vi "Main.vi"() -> ()   [LabVIEW 2019]
doc: "Use this template to build a simple state machine design pattern. Each state executes code and determines which state to transition to."
uses:
  controls/State.ctl
  controls/Data.ctl
  19129ee7-2167-46f5-94c7-6c94359de5af.vi
  97020e74-c88b-4e28-9d88-861c136ab0ec.vi
  3c8d42af-6aab-4c71-abb2-08a78789fadc.vi
  e1166f26-e34e-4867-bf64-0f2b722d0543.vi
  bf01d7cc-2561-4f26-92a1-0952a6f05fec.vi
  86db6c87-178c-447d-b6dd-f69cb95457e9.vi
  da4ff3ae-118d-429f-89dd-6d204435764b.vi
  6bd7f036-247f-456b-9d75-44be66b4905f.vi
  945257d8-b946-4064-894d-b06f0ac42300.vi
  0b4e00a9-1667-44d7-8672-90e7e78b343c.vi
  5caef232-9b1d-433d-a0d0-0ef1dc360dc2.vi
  663dc032-b822-4887-a4ac-48573fd9169f.vi
  31c5358b-7e5d-432a-9607-e566ad1521c2.vi
  71a76362-c902-4af5-9e49-a2a977d014ca.vi
  ba676aeb-3a27-434e-9a7e-9afe782587b5.vi
  86c68439-f49f-4d4b-9d68-38f5b6fe5469.vi
  25f27556-7067-46a7-b570-d4658504531b.vi
  eab5cf03-8b77-4dda-81a4-4f254e97d93e.vi
  fdccc99e-0b2a-4617-a728-f0ef31699cf6.vi
  a5814f98-bddc-4bba-a6ba-c09daa687ff9.vi
panel:
  out "Cycle":u64
  out "Result":bool
  out "LED_OFF":bool
  out "LED_ON":bool
  out "Fan_On (rpm)":dbl
  out "FAN_OFF":bool
  out "FAN_ON":bool
  out "Time_Out":i8
  out "Status":string
  out "Motor_Lock":bool
  out "CAN_ID":u32 format="%.0x"
  out "Motor_Unlock":bool
  out "Rx_DATA":u8[](array[numeric]) format="%x"
  in  "Rx_ID":u32=1968
  out "Tx_DATA":u8[](array[numeric])
  out "Tx_ID":u32=1952
  out "CAN_Tx":bool
  in  "Stop":bool
  in  "TPCANMsg To Write":T1 {"ID" format="%x"; "MSGTYPE" items=["STATUS"=128, "EXTENDED"=2, "RTR"=1, "DATA MSG"=0]; "aDATA" format="%x"}
  out "Last Error":string
  in  "Start":bool
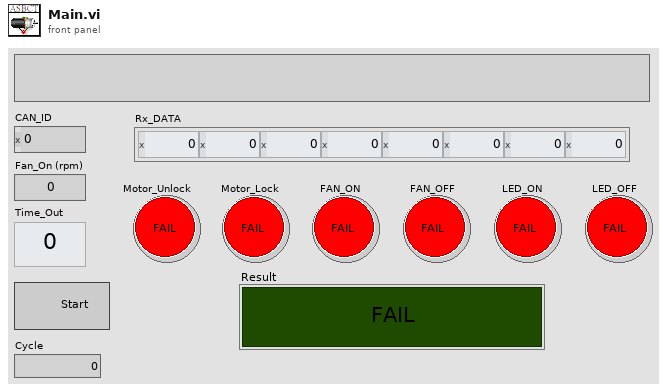
[diagram p1: front panel]
types:
  T1 = cluster{"ID":u32, "MSGTYPE":u8, "LEN":u8, "aDATA":u8[]}
  T2 = typedef "Data.ctl" = cluster{"Status":string, "Cycle":u64, "Result":bool[]}
  T3 = typedef "State.ctl" = enum16{"Initialize", "Wait for Event", "Motor_Remove", "Motor_Insert", "Fan_On", "Fan_Off", "Led_On", "Led_Off"}
  T4 = typedef "PCAN_ERROR.ctl" = i32
  T5 = cluster{"Is Warning":bool, "Is Error":bool, "Message":string}
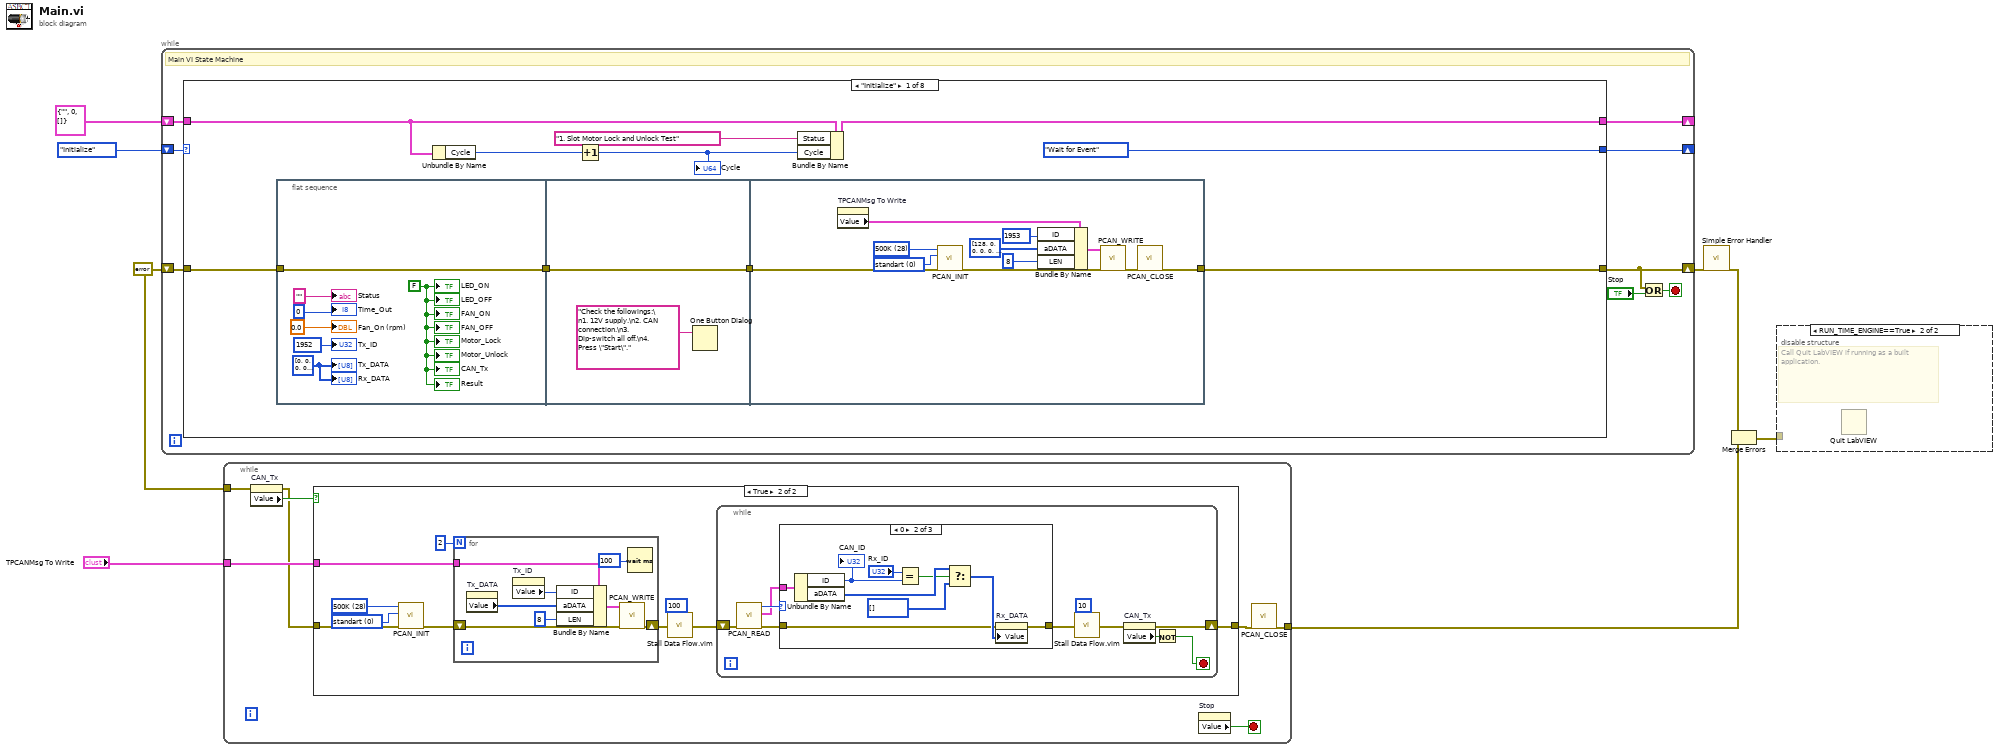
[diagram p0: block diagram]
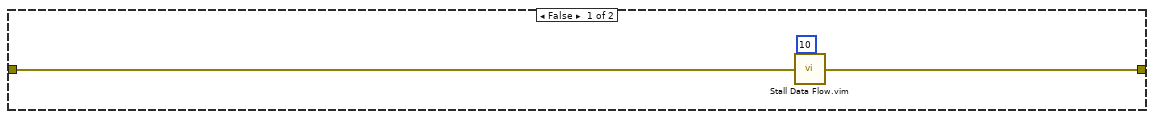
[diagram p2: hidden frame]
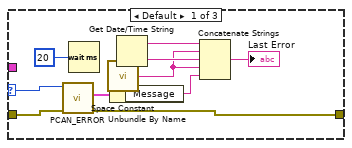
[diagram p3: hidden frame]
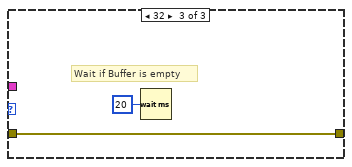
[diagram p4: hidden frame]
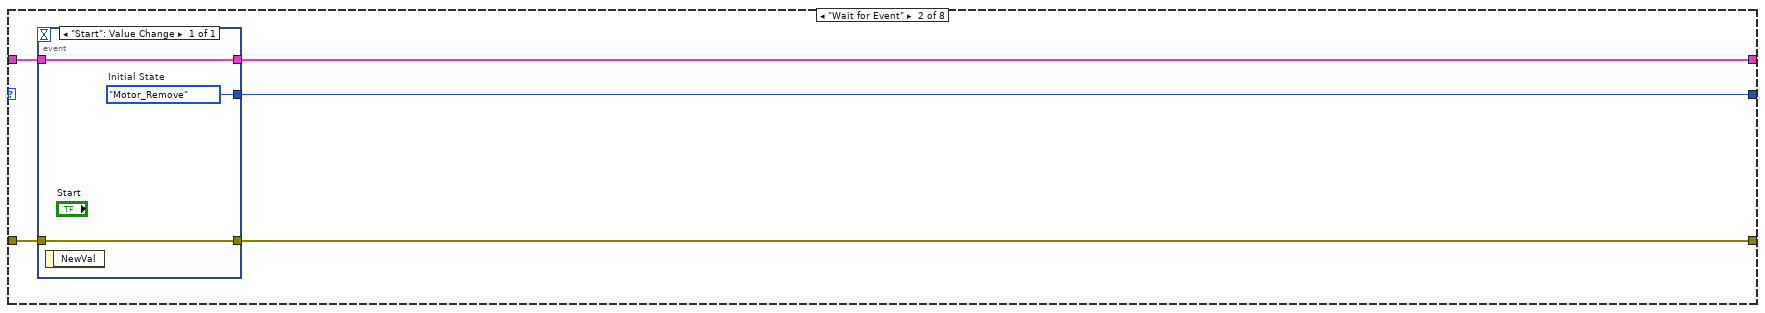
[diagram p6: hidden frame]
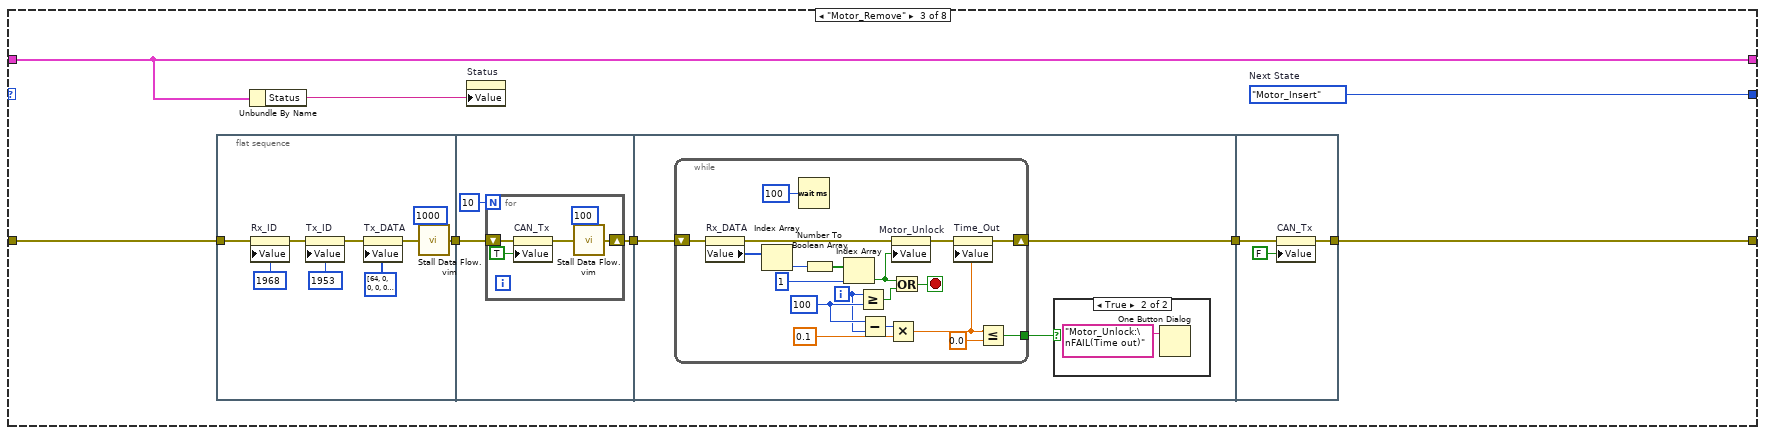
[diagram p7: hidden frame]
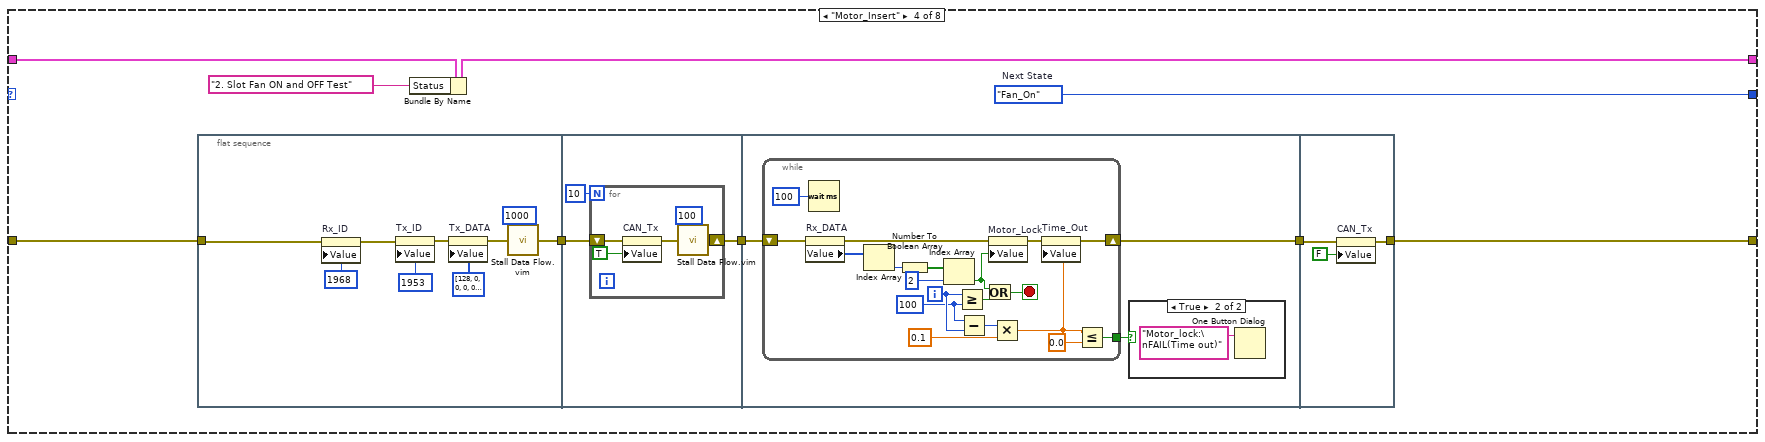
[diagram p9: hidden frame]
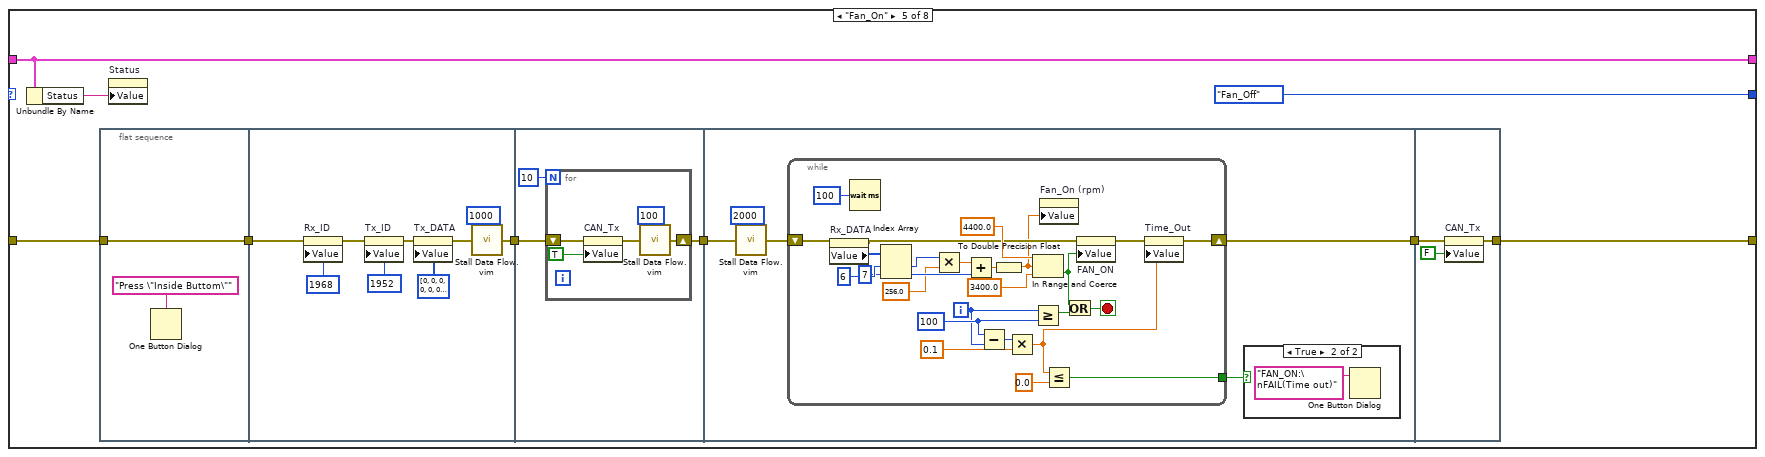
[diagram p11: hidden frame]
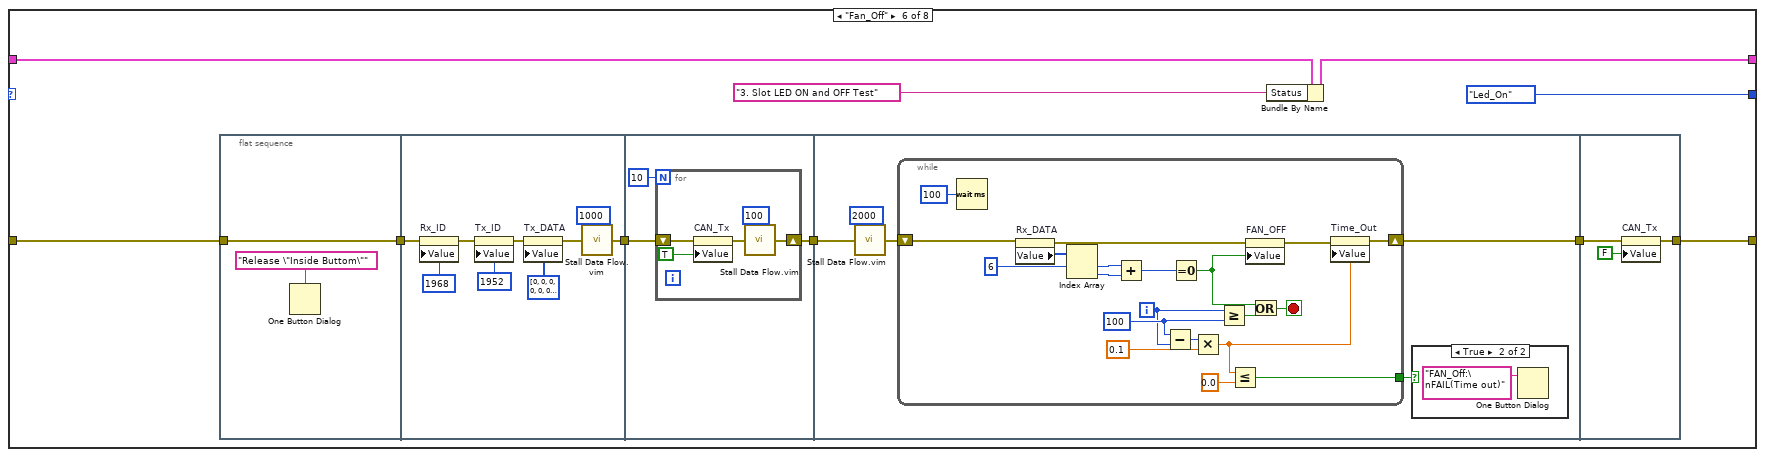
[diagram p13: hidden frame]
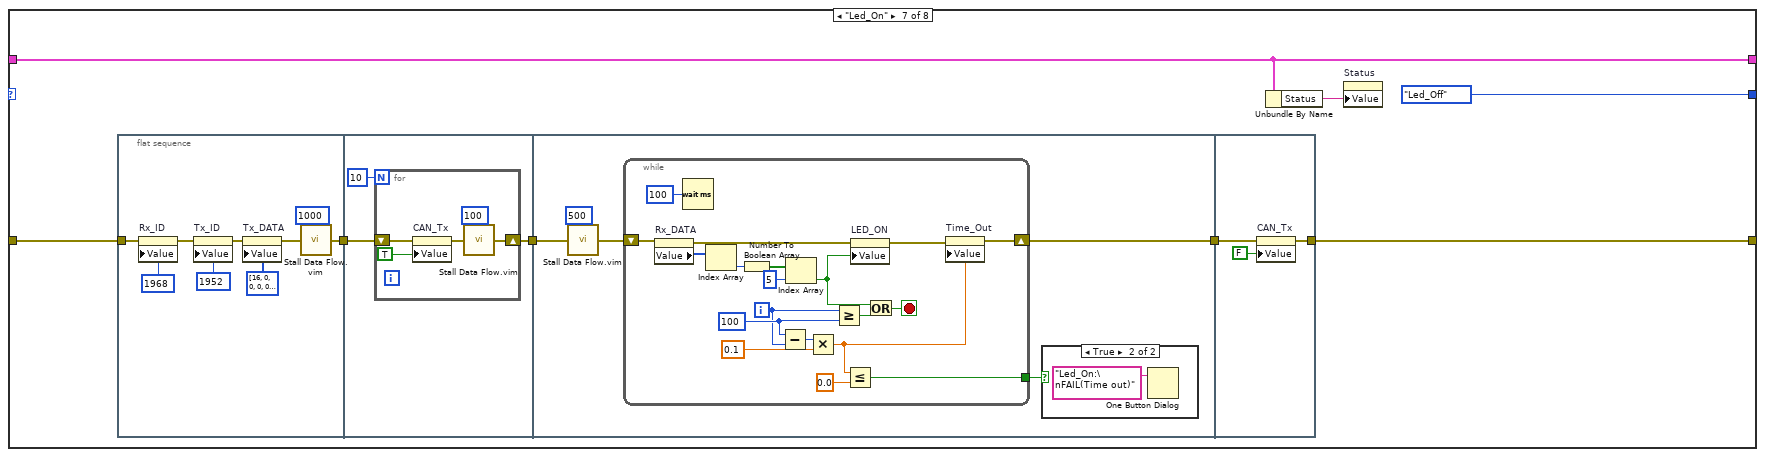
[diagram p15: hidden frame]
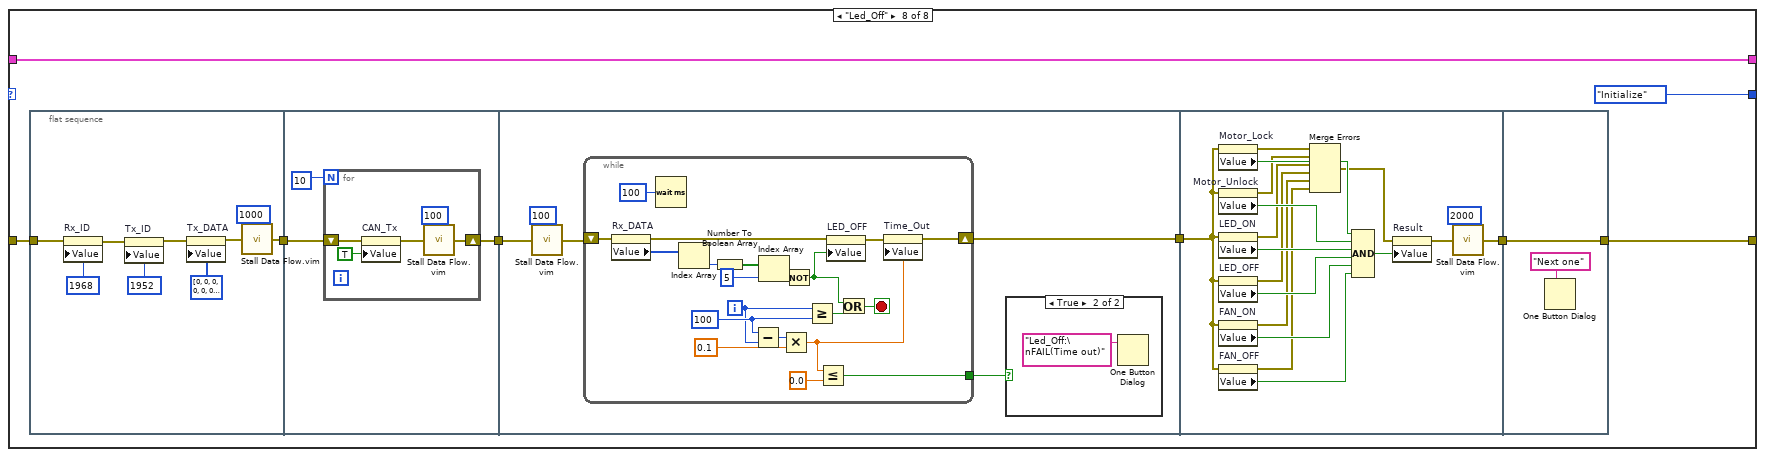
[diagram p17: hidden frame]
diagram:
  w1 = errorcluster {"status"=FALSE, "code"=0, "source"=""} ("error constant")
  n1 = while {
    shift-right: [w10] -> _
    shift-left: State."Initialize" ("Initial State") -> [w11]
    shift-right: [w15] -> _
    shift-left: T2 {"Status"="", "Cycle"=0, "Result"=[]} ("Data") -> [w16]
    shift-right: [w12] -> w7
    shift-left: w1 -> [w14]
    stop <- w13 stop-if-true
    # "Main VI State Machine"
    n2 = case shown="\"Initialize\"" w11 {
      tunnel: [State."Wait for Event" ("Next") w47 w62 w114 State."Fan_Off" ("(Value Not Used)") State."Led_On" ("(Value Not Used)") State."Led_Off" ("(Value Not Used)") State."Initialize" ("(Value Not Used)")] -> w10
      tunnel: w16 -> [w19 w51 w60 w111 w162 w225 w280 w332]
      tunnel: [w26 w50 w60 w110 w162 w224 w280 w332] -> w15
      tunnel: w14 -> [w23 w49 w61 w112 w164 w228 w284 w337]
      tunnel: [w24 w48 w55 w106 w158 w222 w281 w338] -> w12
      frame "Initialize" {
        # "Initialize - Initialize the application."
        n3 = flat-sequence {
          tunnel: w23 -> [w33]
          tunnel: [w33] -> w21
          tunnel: w21 -> [w35]
          tunnel: [w35] -> w20
          tunnel: [w36] -> w24
          tunnel: w20 -> [w44]
          frame #0 {
            w28 = u8[] [0, 0, 0, 0, 0, 0, 0, 0] ("aDATA")
            w27 = FALSE ("Replace_Me_Boolean")
            "Time_Out" <- i8 0 ("Time_Out")
            "Status" <- "" ("Status")
            "Fan_On (rpm)" <- 0.0 ("FAN(rpm)")
            "CAN_Tx" <- w27
            "Motor_Unlock" <- w27
            "Motor_Lock" <- w27
            "FAN_ON" <- w27
            "FAN_OFF" <- w27
            "LED_ON" <- w27
            "LED_OFF" <- w27
            "Tx_ID" <- u32 1952 ("ID")
            "Tx_DATA" <- w28
            "Rx_DATA" <- w28
            "Result" <- w27
          }
          frame #1 {
            n4 = One Button Dialog(message="Check the followings:\n1. 12V supply.\n2. CAN connection.\n3. Dip-switch all off.\n4. Press \"Start\".") -> ()  [unwired: 1 in, 1 out]
          }
          frame #2 {
            w46 = 0 items=["standart", "extended"] ("type")
            w45 = u16 28 items=["1M"=20, "500K"=28, "250K"=284, "125K"=796, "100K"=17199, "50K"=18223, "20K"=21295, "10K"=26415, "5K"=32639] ("baud")
            n5 = property on="TPCANMsg To Write" class="Clust (strict)"() -> ("Value"=w42:T1)  [unwired: 2 in, 2 out]
            n6 = call "PCAN_INIT.vi"("error in (no error)"=w44, "Msg Type"=w46, "BTR0BTR1"=w45) -> ("error out"=w40:errorcluster)  [unwired: 1 in, 7 out]
            n7 = Bundle By Name(cluster=w42, "ID"=u32 1953, "aDATA"=u8[] [128, 0, 0, 0, 0, 0, 0, 0], "LEN"=u8 8) -> (w41:T1)
            n8 = call "PCAN_WRITE.vi"("error in (no error)"=w40, "TPCANMsg"=w41) -> ("error out"=w37:errorcluster)  [unwired: 1 in, 8 out]
            n9 = call "PCAN_CLOSE.vi"("error in (no error)"=w37) -> ("error out"=w36:errorcluster)  [unwired: 10 out]
          }
        }
        n10 = Unbundle By Name(w19) -> ("Cycle"=w18:u64)
        n11 = Increment(x=w18) -> (x+1=w17:u64)
        "Cycle" <- w17
        n12 = Bundle By Name(cluster=w19, "Status"="1. Slot Motor Lock and Unlock Test" ("Running User State 1"), "Cycle"=w17) -> (w26:T2)
      }
      frame "Wait for Event" {
        # "Wait for Event - Use an Event Structure to monitor the user interface for events that run different states of the state machine."
        n13 = event shown="[0] \"Start\": Value Change" {
          selector: _ -> [_]
          dyn-events: _ -> [_]
          timeout: _ -> [_]
          tunnel: [w53] -> w47
          tunnel: w51 -> [w52]
          tunnel: [w52] -> w50
          tunnel: w49 -> [w54]
          tunnel: [w54] -> w48
          event "Start": Value Change {
            w53 = State."Motor_Remove"  # Initial State
            n14 = event-data() -> ()  [unwired: 1 in, 1 out]
          }
        }
      }
      frame "Motor_Remove" {
        w62 = State."Motor_Insert"  # Next State
        # "User State 1 - Replace this state with functionality for your own application."
        n15 = flat-sequence {
          tunnel: w61 -> [w63]
          tunnel: [w66] -> w57
          tunnel: w57 -> [w74]
          tunnel: [w72] -> w56
          tunnel: [w82] -> w58
          tunnel: w56 -> [w80]
          tunnel: [w104] -> w55
          tunnel: w58 -> [w105]
          frame #0 {
            n16 = property on="Rx_ID" class="DigNum (strict)"(error in=w63, "Value"=u32 1968 ("Rx_ID")) -> (error out=w64:errorcluster)  [unwired: 1 in, 1 out]
            n17 = property on="Tx_ID" class="DigNum (strict)"(error in=w64, "Value"=u32 1953 ("ID")) -> (error out=w69:errorcluster)  [unwired: 1 in, 1 out]
            n18 = property on="Tx_DATA" class="Arr (strict)"(error in=w69, "Value"=u8[] [64, 0, 0, 0, 0, 0, 0, 0] ("aDATA")) -> (error out=w67:errorcluster)  [unwired: 1 in, 1 out]
            n19 = call "Stall Data Flow.vim"("value in"=w67, "milliseconds to wait"=u32 1000) -> ("value out"=w66:errorcluster)  [unwired: 1 out]
          }
          frame #1 {
            n20 = for {
              N: 10 -> [_]
              shift-right: [w76] -> w72
              shift-left: w74 -> [w79]
              n21 = property on="CAN_Tx" class="Bool (strict)"(error in=w79, "Value"=TRUE ("CAN_Tx")) -> (error out=w75:errorcluster)  [unwired: 1 in, 1 out]
              n22 = call "Stall Data Flow.vim"("value in"=w75, "milliseconds to wait"=u32 100) -> ("value out"=w76:errorcluster)  [unwired: 1 out]
            }
          }
          frame #2 {
            n23 = while {
              shift-right: [w92] -> w82
              shift-left: w80 -> [w88]
              tunnel: [w89] -> w81
              i -> [w96]
              stop <- w98 stop-if-true
              w97 = 100
              n24 = property on="Rx_DATA" class="Arr (strict)"(error in=w88) -> (error out=w100:errorcluster, "Value"=w102:u8[])  [unwired: 1 in, 1 out]
              n25 = Index Array(array=w102) -> (element=w85:u8)  [unwired: 1 in]
              n26 = Wait (ms)(milliseconds to wait=u32 100) -> ()  [unwired: 1 out]
              n27 = Number To Boolean Array(number=w85) -> (Boolean array=w86:bool[])
              n28 = Index Array(array=w86, index=1) -> (element=w84:bool)
              n29 = Greater Or Equal?(x=w96, y=w97) -> (x >= y?=w99:bool)
              n30 = Subtract(x=w97, y=w96) -> (x-y=w95:i32)
              n31 = Multiply(x=w95, y=0.1) -> (x*y=w91:dbl)
              n32 = property on="Motor_Unlock" class="Bool (strict)"(error in=w100, "Value"=w84) -> (error out=w93:errorcluster)  [unwired: 1 in, 1 out]
              n33 = Or(x=w84, y=w99) -> (x .or. y?=w98:bool)
              n34 = property on="Time_Out" class="DigNum (strict)"(error in=w93, "Value"=w91) -> (error out=w92:errorcluster)  [unwired: 1 in, 1 out]
              n35 = Less Or Equal?(x=w91, y=0.0) -> (x <= y?=w89:bool)
            }
            n36 = case shown="True" w81 {
              frame False {
              }
              frame True {
                n37 = One Button Dialog(message="Motor_Unlock:\nFAIL(Time out)") -> ()  [unwired: 1 in, 1 out]
              }
            }
          }
          frame #3 {
            n38 = property on="CAN_Tx" class="Bool (strict)"(error in=w105, "Value"=FALSE ("CAN_Tx")) -> (error out=w104:errorcluster)  [unwired: 1 in, 1 out]
          }
        }
        n39 = Unbundle By Name(w60) -> ("Status"=w59:string)
        n40 = property on="Status" class="Str"("Value"=w59) -> ()  [unwired: 2 in, 2 out]
      }
      frame "Motor_Insert" {
        w114 = State."Fan_On"  # Next State
        # "User State 2 - Replace this state with functionality for your own application."
        n41 = flat-sequence {
          tunnel: w112 -> [w115]
          tunnel: [w118] -> w113
          tunnel: w113 -> [w126]
          tunnel: [w124] -> w107
          tunnel: [w134] -> w108
          tunnel: w107 -> [w132]
          tunnel: [w156] -> w106
          tunnel: w108 -> [w157]
          frame #0 {
            n42 = property on="Rx_ID" class="DigNum (strict)"(error in=w115, "Value"=u32 1968 ("Rx_ID")) -> (error out=w116:errorcluster)  [unwired: 1 in, 1 out]
            n43 = property on="Tx_ID" class="DigNum (strict)"(error in=w116, "Value"=u32 1953 ("ID")) -> (error out=w121:errorcluster)  [unwired: 1 in, 1 out]
            n44 = property on="Tx_DATA" class="Arr (strict)"(error in=w121, "Value"=u8[] [128, 0, 0, 0, 0, 0, 0, 0] ("aDATA")) -> (error out=w119:errorcluster)  [unwired: 1 in, 1 out]
            n45 = call "Stall Data Flow.vim"("value in"=w119, "milliseconds to wait"=u32 1000) -> ("value out"=w118:errorcluster)  [unwired: 1 out]
          }
          frame #1 {
            n46 = for {
              N: 10 -> [_]
              shift-right: [w127] -> w124
              shift-left: w126 -> [w131]
              n47 = property on="CAN_Tx" class="Bool (strict)"(error in=w131, "Value"=TRUE ("CAN_Tx")) -> (error out=w128:errorcluster)  [unwired: 1 in, 1 out]
              n48 = call "Stall Data Flow.vim"("value in"=w128, "milliseconds to wait"=u32 100) -> ("value out"=w127:errorcluster)  [unwired: 1 out]
            }
          }
          frame #2 {
            n49 = while {
              shift-right: [w143] -> w134
              shift-left: w132 -> [w140]
              tunnel: [w145] -> w133
              i -> [w149]
              stop <- w150 stop-if-true
              w141 = 100
              n50 = property on="Rx_DATA" class="Arr (strict)"(error in=w140) -> (error out=w152:errorcluster, "Value"=w153:u8[])  [unwired: 1 in, 1 out]
              n51 = Wait (ms)(milliseconds to wait=u32 100) -> ()  [unwired: 1 out]
              n52 = Index Array(array=w153) -> (element=w137:u8)  [unwired: 1 in]
              n53 = Number To Boolean Array(number=w137) -> (Boolean array=w138:bool[])
              n54 = Index Array(array=w138, index=2) -> (element=w136:bool)
              n55 = Greater Or Equal?(x=w149, y=w141) -> (x >= y?=w151:bool)
              n56 = Subtract(x=w141, y=w149) -> (x-y=w148:i32)
              n57 = Or(x=w136, y=w151) -> (x .or. y?=w150:bool)
              n58 = property on="Motor_Lock" class="Bool (strict)"(error in=w152, "Value"=w136) -> (error out=w144:errorcluster)  [unwired: 1 in, 1 out]
              n59 = Multiply(x=w148, y=0.1) -> (x*y=w142:dbl)
              n60 = property on="Time_Out" class="DigNum (strict)"(error in=w144, "Value"=w142) -> (error out=w143:errorcluster)  [unwired: 1 in, 1 out]
              n61 = Less Or Equal?(x=w142, y=0.0) -> (x <= y?=w145:bool)
            }
            n62 = case shown="True" w133 {
              frame False {
              }
              frame True {
                n63 = One Button Dialog(message="Motor_lock:\nFAIL(Time out)") -> ()  [unwired: 1 in, 1 out]
              }
            }
          }
          frame #3 {
            n64 = property on="CAN_Tx" class="Bool (strict)"(error in=w157, "Value"=FALSE ("CAN_Tx")) -> (error out=w156:errorcluster)  [unwired: 1 in, 1 out]
          }
        }
        n65 = Bundle By Name(cluster=w111, "Status"="2. Slot Fan ON and OFF Test") -> (w110:T2)
      }
      frame "Fan_On" {
        n66 = Unbundle By Name(w162) -> ("Status"=w161:string)
        n67 = flat-sequence {
          tunnel: w164 -> [w168]
          tunnel: [w168] -> w159
          tunnel: [w172] -> w166
          tunnel: w159 -> [w169]
          tunnel: w166 -> [w180]
          tunnel: [w179] -> w165
          tunnel: w165 -> [w187]
          tunnel: [w190] -> w160
          tunnel: [w219] -> w158
          tunnel: w160 -> [w220]
          frame #0 {
            n68 = One Button Dialog(message="Press \"Inside Buttom\"") -> ()  [unwired: 1 in, 1 out]
          }
          frame #1 {
            n69 = property on="Rx_ID" class="DigNum (strict)"(error in=w169, "Value"=u32 1968 ("Rx_ID")) -> (error out=w170:errorcluster)  [unwired: 1 in, 1 out]
            n70 = property on="Tx_ID" class="DigNum (strict)"(error in=w170, "Value"=u32 1952 ("ID")) -> (error out=w176:errorcluster)  [unwired: 1 in, 1 out]
            n71 = property on="Tx_DATA" class="Arr (strict)"(error in=w176, "Value"=u8[] [0, 0, 0, 0, 0, 0, 128, 0] ("aDATA")) -> (error out=w173:errorcluster)  [unwired: 1 in, 1 out]
            n72 = call "Stall Data Flow.vim"("value in"=w173, "milliseconds to wait"=u32 1000) -> ("value out"=w172:errorcluster)  [unwired: 1 out]
          }
          frame #2 {
            n73 = for {
              N: 10 -> [_]
              shift-right: [w181] -> w179
              shift-left: w180 -> [w185]
              n74 = property on="CAN_Tx" class="Bool (strict)"(error in=w185, "Value"=TRUE ("CAN_Tx")) -> (error out=w182:errorcluster)  [unwired: 1 in, 1 out]
              n75 = call "Stall Data Flow.vim"("value in"=w182, "milliseconds to wait"=u32 100) -> ("value out"=w181:errorcluster)  [unwired: 1 out]
            }
          }
          frame #3 {
            n76 = call "Stall Data Flow.vim"("value in"=w187, "milliseconds to wait"=u32 2000) -> ("value out"=w186:errorcluster)  [unwired: 1 out]
            n77 = while {
              shift-right: [w195] -> w190
              shift-left: w186 -> [w192]
              tunnel: [w210] -> w189
              i -> [w214]
              stop <- w216 stop-if-true
              w215 = 100
              n78 = property on="Rx_DATA" class="Arr (strict)"(error in=w192) -> (error out=w202:errorcluster, "Value"=w209:u8[])  [unwired: 1 in, 1 out]
              n79 = Wait (ms)(milliseconds to wait=u32 100) -> ()  [unwired: 1 out]
              n80 = Index Array(array=w209, index #1=6 ("index"), index #2=7 ("index")) -> (element #1=w198:u8, element #2=w207:u8)
              n81 = Multiply(x=w198, y=256.0 ("lower limit")) -> (x*y=w199:dbl)
              n82 = Add(x=w199, y=w207) -> (x+y=w206:dbl)
              n83 = Subtract(x=w215, y=w214) -> (x-y=w213:i32)
              n84 = To Double Precision Float(number=w206) -> (double precision float=w200:dbl)
              n85 = Multiply(x=w213, y=0.1) -> (x*y=w194:dbl)
              n86 = In Range and Coerce(upper limit=4400.0, x=w200, lower limit=3400.0) -> (In Range?=w201:bool)  [unwired: 1 out]
              n87 = Greater Or Equal?(x=w214, y=w215) -> (x >= y?=w203:bool)
              n88 = property on="Fan_On (rpm)" class="DigNum (strict)"("Value"=w200) -> ()  [unwired: 2 in, 2 out]
              n89 = Less Or Equal?(x=w194, y=0.0) -> (x <= y?=w210:bool)
              n90 = Or(x=w201, y=w203) -> (x .or. y?=w216:bool)
              n91 = property on="FAN_ON" class="Bool (strict)"(error in=w202, "Value"=w201) -> (error out=w196:errorcluster)  [unwired: 1 in, 1 out]
              n92 = property on="Time_Out" class="DigNum (strict)"(error in=w196, "Value"=w194) -> (error out=w195:errorcluster)  [unwired: 1 in, 1 out]
            }
            n93 = case shown="True" w189 {
              frame False {
              }
              frame True {
                n94 = One Button Dialog(message="FAN_ON:\nFAIL(Time out)") -> ()  [unwired: 1 in, 1 out]
              }
            }
          }
          frame #4 {
            n95 = property on="CAN_Tx" class="Bool (strict)"(error in=w220, "Value"=FALSE ("CAN_Tx")) -> (error out=w219:errorcluster)  [unwired: 1 in, 1 out]
          }
        }
        n96 = property on="Status" class="Str"("Value"=w161) -> ()  [unwired: 2 in, 2 out]
      }
      frame "Fan_Off" {
        n97 = flat-sequence {
          tunnel: w228 -> [w232]
          tunnel: [w232] -> w221
          tunnel: [w237] -> w230
          tunnel: w221 -> [w233]
          tunnel: w230 -> [w244]
          tunnel: [w243] -> w229
          tunnel: w229 -> [w251]
          tunnel: [w254] -> w226
          tunnel: [w277] -> w222
          tunnel: w226 -> [w278]
          frame #0 {
            n98 = One Button Dialog(message="Release \"Inside Buttom\"") -> ()  [unwired: 1 in, 1 out]
          }
          frame #1 {
            n99 = property on="Rx_ID" class="DigNum (strict)"(error in=w233, "Value"=u32 1968 ("Rx_ID")) -> (error out=w234:errorcluster)  [unwired: 1 in, 1 out]
            n100 = property on="Tx_ID" class="DigNum (strict)"(error in=w234, "Value"=u32 1952 ("ID")) -> (error out=w240:errorcluster)  [unwired: 1 in, 1 out]
            n101 = property on="Tx_DATA" class="Arr (strict)"(error in=w240, "Value"=u8[] [0, 0, 0, 0, 0, 0, 0, 0] ("aDATA")) -> (error out=w238:errorcluster)  [unwired: 1 in, 1 out]
            n102 = call "Stall Data Flow.vim"("value in"=w238, "milliseconds to wait"=u32 1000) -> ("value out"=w237:errorcluster)  [unwired: 1 out]
          }
          frame #2 {
            n103 = for {
              N: 10 -> [_]
              shift-right: [w245] -> w243
              shift-left: w244 -> [w249]
              n104 = property on="CAN_Tx" class="Bool (strict)"(error in=w249, "Value"=TRUE ("CAN_Tx")) -> (error out=w246:errorcluster)  [unwired: 1 in, 1 out]
              n105 = call "Stall Data Flow.vim"("value in"=w246, "milliseconds to wait"=u32 100) -> ("value out"=w245:errorcluster)  [unwired: 1 out]
            }
          }
          frame #3 {
            n106 = call "Stall Data Flow.vim"("value in"=w251, "milliseconds to wait"=u32 2000) -> ("value out"=w250:errorcluster)  [unwired: 1 out]
            n107 = while {
              shift-right: [w264] -> w254
              shift-left: w250 -> [w257]
              tunnel: [w268] -> w253
              i -> [w272]
              stop <- w274 stop-if-true
              w273 = 100
              n108 = Wait (ms)(milliseconds to wait=u32 100) -> ()  [unwired: 1 out]
              n109 = property on="Rx_DATA" class="Arr (strict)"(error in=w257) -> (error out=w259:errorcluster, "Value"=w267:u8[])  [unwired: 1 in, 1 out]
              n110 = Index Array(array=w267, index #1=6 ("index")) -> (element #1=w262:u8, element #2=w261:u8)  [unwired: 1 in]
              n111 = Add(x=w262, y=w261) -> (x+y=w260:u8)
              n112 = Subtract(x=w273, y=w272) -> (x-y=w271:i32)
              n113 = Equal To 0?(x=w260) -> (x = 0?=w256:bool)
              n114 = Multiply(x=w271, y=0.1) -> (x*y=w263:dbl)
              n115 = Greater Or Equal?(x=w272, y=w273) -> (x >= y?=w265:bool)
              n116 = Less Or Equal?(x=w263, y=0.0) -> (x <= y?=w268:bool)
              n117 = property on="FAN_OFF" class="Bool (strict)"(error in=w259, "Value"=w256) -> (error out=w258:errorcluster)  [unwired: 1 in, 1 out]
              n118 = Or(x=w256, y=w265) -> (x .or. y?=w274:bool)
              n119 = property on="Time_Out" class="DigNum (strict)"(error in=w258, "Value"=w263) -> (error out=w264:errorcluster)  [unwired: 1 in, 1 out]
            }
            n120 = case shown="True" w253 {
              frame False {
              }
              frame True {
                n121 = One Button Dialog(message="FAN_Off:\nFAIL(Time out)") -> ()  [unwired: 1 in, 1 out]
              }
            }
          }
          frame #4 {
            n122 = property on="CAN_Tx" class="Bool (strict)"(error in=w278, "Value"=FALSE ("CAN_Tx")) -> (error out=w277:errorcluster)  [unwired: 1 in, 1 out]
          }
        }
        n123 = Bundle By Name(cluster=w225, "Status"="3. Slot LED ON and OFF Test") -> (w224:T2)
      }
      frame "Led_On" {
        n124 = flat-sequence {
          tunnel: [w291] -> w286
          tunnel: w284 -> [w288]
          tunnel: w286 -> [w298]
          tunnel: [w297] -> w285
          tunnel: w285 -> [w305]
          tunnel: [w308] -> w282
          tunnel: [w330] -> w281
          tunnel: w282 -> [w331]
          frame #0 {
            n125 = property on="Rx_ID" class="DigNum (strict)"(error in=w288, "Value"=u32 1968 ("Rx_ID")) -> (error out=w289:errorcluster)  [unwired: 1 in, 1 out]
            n126 = property on="Tx_ID" class="DigNum (strict)"(error in=w289, "Value"=u32 1952 ("ID")) -> (error out=w294:errorcluster)  [unwired: 1 in, 1 out]
            n127 = property on="Tx_DATA" class="Arr (strict)"(error in=w294, "Value"=u8[] [16, 0, 0, 0, 0, 0, 0, 0] ("aDATA")) -> (error out=w292:errorcluster)  [unwired: 1 in, 1 out]
            n128 = call "Stall Data Flow.vim"("value in"=w292, "milliseconds to wait"=u32 1000) -> ("value out"=w291:errorcluster)  [unwired: 1 out]
          }
          frame #1 {
            n129 = for {
              N: 10 -> [_]
              shift-right: [w299] -> w297
              shift-left: w298 -> [w303]
              n130 = property on="CAN_Tx" class="Bool (strict)"(error in=w303, "Value"=TRUE ("CAN_Tx")) -> (error out=w300:errorcluster)  [unwired: 1 in, 1 out]
              n131 = call "Stall Data Flow.vim"("value in"=w300, "milliseconds to wait"=u32 100) -> ("value out"=w299:errorcluster)  [unwired: 1 out]
            }
          }
          frame #2 {
            n132 = call "Stall Data Flow.vim"("value in"=w305, "milliseconds to wait"=u32 500) -> ("value out"=w304:errorcluster)  [unwired: 1 out]
            n133 = while {
              shift-right: [w318] -> w308
              shift-left: w304 -> [w316]
              tunnel: [w321] -> w307
              i -> [w325]
              stop <- w327 stop-if-true
              w326 = 100
              n134 = property on="Rx_DATA" class="Arr (strict)"(error in=w316) -> (error out=w315:errorcluster, "Value"=w320:u8[])  [unwired: 1 in, 1 out]
              n135 = Wait (ms)(milliseconds to wait=u32 100) -> ()  [unwired: 1 out]
              n136 = Index Array(array=w320) -> (element=w313:u8)  [unwired: 1 in]
              n137 = Number To Boolean Array(number=w313) -> (Boolean array=w311:bool[])
              n138 = Subtract(x=w326, y=w325) -> (x-y=w324:i32)
              n139 = Index Array(array=w311, index=5) -> (element=w310:bool)
              n140 = Multiply(x=w324, y=0.1) -> (x*y=w317:dbl)
              n141 = Greater Or Equal?(x=w325, y=w326) -> (x >= y?=w319:bool)
              n142 = Less Or Equal?(x=w317, y=0.0) -> (x <= y?=w321:bool)
              n143 = property on="LED_ON" class="Bool (strict)"(error in=w315, "Value"=w310) -> (error out=w314:errorcluster)  [unwired: 1 in, 1 out]
              n144 = Or(x=w310, y=w319) -> (x .or. y?=w327:bool)
              n145 = property on="Time_Out" class="DigNum (strict)"(error in=w314, "Value"=w317) -> (error out=w318:errorcluster)  [unwired: 1 in, 1 out]
            }
            n146 = case shown="True" w307 {
              frame False {
              }
              frame True {
                n147 = One Button Dialog(message="Led_On:\nFAIL(Time out)") -> ()  [unwired: 1 in, 1 out]
              }
            }
          }
          frame #3 {
            n148 = property on="CAN_Tx" class="Bool (strict)"(error in=w331, "Value"=FALSE ("CAN_Tx")) -> (error out=w330:errorcluster)  [unwired: 1 in, 1 out]
          }
        }
        n149 = Unbundle By Name(w280) -> ("Status"=w279:string)
        n150 = property on="Status" class="Str"("Value"=w279) -> ()  [unwired: 2 in, 2 out]
      }
      frame "Led_Off" {
        n151 = flat-sequence {
          tunnel: w337 -> [w348]
          tunnel: [w340] -> w334
          tunnel: w334 -> [w350]
          tunnel: [w349] -> w333
          tunnel: w333 -> [w358]
          tunnel: [w360] -> w336
          tunnel: w336 -> [w400]
          tunnel: [w384] -> w335
          tunnel: [w402] -> w338
          tunnel: w335 -> [w402]
          frame #0 {
            n152 = property on="Rx_ID" class="DigNum (strict)"(error in=w348, "Value"=u32 1968 ("Rx_ID")) -> (error out=w346:errorcluster)  [unwired: 1 in, 1 out]
            n153 = property on="Tx_ID" class="DigNum (strict)"(error in=w346, "Value"=u32 1952 ("ID")) -> (error out=w344:errorcluster)  [unwired: 1 in, 1 out]
            n154 = property on="Tx_DATA" class="Arr (strict)"(error in=w344, "Value"=u8[] [0, 0, 0, 0, 0, 0, 0, 0] ("aDATA")) -> (error out=w341:errorcluster)  [unwired: 1 in, 1 out]
            n155 = call "Stall Data Flow.vim"("value in"=w341, "milliseconds to wait"=u32 1000) -> ("value out"=w340:errorcluster)  [unwired: 1 out]
          }
          frame #1 {
            n156 = for {
              N: 10 -> [_]
              shift-right: [w353] -> w349
              shift-left: w350 -> [w355]
              n157 = property on="CAN_Tx" class="Bool (strict)"(error in=w355, "Value"=TRUE ("CAN_Tx")) -> (error out=w354:errorcluster)  [unwired: 1 in, 1 out]
              n158 = call "Stall Data Flow.vim"("value in"=w354, "milliseconds to wait"=u32 100) -> ("value out"=w353:errorcluster)  [unwired: 1 out]
            }
          }
          frame #2 {
            n159 = call "Stall Data Flow.vim"("value in"=w358, "milliseconds to wait"=u32 100) -> ("value out"=w357:errorcluster)  [unwired: 1 out]
            n160 = while {
              shift-right: [w368] -> w360
              shift-left: w357 -> [w370]
              tunnel: [w375] -> w361
              i -> [w379]
              stop <- w381 stop-if-true
              w380 = 100
              n161 = property on="Rx_DATA" class="Arr (strict)"(error in=w370) -> (error out=w366:errorcluster, "Value"=w369:u8[])  [unwired: 1 in, 1 out]
              n162 = Wait (ms)(milliseconds to wait=u32 100) -> ()  [unwired: 1 out]
              n163 = Index Array(array=w369) -> (element=w373:u8)  [unwired: 1 in]
              n164 = Number To Boolean Array(number=w373) -> (Boolean array=w371:bool[])
              n165 = Subtract(x=w380, y=w379) -> (x-y=w378:i32)
              n166 = Index Array(array=w371, index=5) -> (element=w364:bool)
              n167 = Multiply(x=w378, y=0.1) -> (x*y=w367:dbl)
              n168 = Not(x=w364) -> (.not. x?=w363:bool)
              n169 = Greater Or Equal?(x=w379, y=w380) -> (x >= y?=w374:bool)
              n170 = Less Or Equal?(x=w367, y=0.0) -> (x <= y?=w375:bool)
              n171 = property on="LED_OFF" class="Bool (strict)"(error in=w366, "Value"=w363) -> (error out=w365:errorcluster)  [unwired: 1 in, 1 out]
              n172 = Or(x=w363, y=w374) -> (x .or. y?=w381:bool)
              n173 = property on="Time_Out" class="DigNum (strict)"(error in=w365, "Value"=w367) -> (error out=w368:errorcluster)  [unwired: 1 in, 1 out]
            }
            n174 = case shown="True" w361 {
              frame False {
              }
              frame True {
                n175 = One Button Dialog(message="Led_Off:\nFAIL(Time out)") -> ()  [unwired: 1 in, 1 out]
              }
            }
          }
          frame #3 {
            n176 = property on="Motor_Lock" class="Bool (strict)"(error in=w400) -> (error out=w393:errorcluster, "Value"=w399:bool)  [unwired: 1 in, 1 out]
            n177 = property on="Motor_Unlock" class="Bool (strict)"(error in=w400) -> (error out=w392:errorcluster, "Value"=w398:bool)  [unwired: 1 in, 1 out]
            n178 = property on="LED_ON" class="Bool (strict)"(error in=w400) -> (error out=w391:errorcluster, "Value"=w397:bool)  [unwired: 1 in, 1 out]
            n179 = property on="LED_OFF" class="Bool (strict)"(error in=w400) -> (error out=w390:errorcluster, "Value"=w396:bool)  [unwired: 1 in, 1 out]
            n180 = property on="FAN_ON" class="Bool (strict)"(error in=w400) -> (error out=w388:errorcluster, "Value"=w395:bool)  [unwired: 1 in, 1 out]
            n181 = property on="FAN_OFF" class="Bool (strict)"(error in=w400) -> (error out=w389:errorcluster, "Value"=w394:bool)  [unwired: 1 in, 1 out]
            n182 = Merge Errors(w393, w392, w391, w390, w388, w389) -> (w387:errorcluster)
            n183 = Compound Arithmetic op=AND(w399, w398, w397, w396, w395, w394) -> (w383:bool)
            n184 = property on="Result" class="Bool (strict)"(error in=w387, "Value"=w383) -> (error out=w385:errorcluster)  [unwired: 1 in, 1 out]
            n185 = call "Stall Data Flow.vim"("value in"=w385, "milliseconds to wait"=u32 2000) -> ("value out"=w384:errorcluster)  [unwired: 1 out]
          }
          frame #4 {
            n186 = One Button Dialog(message="Next one") -> ()  [unwired: 1 in, 1 out]
          }
        }
      }
    }
    n187 = Or(x=w12, y="Stop") -> (x .or. y?=w13:bool)
  }
  n188 = while {
    tunnel: "TPCANMsg To Write" -> [w409]
    tunnel: [w405] -> w2
    tunnel: w1 -> [w403]
    stop <- w408 stop-if-true
    n189 = property on="CAN_Tx" class="Bool (strict)"(error in=w403) -> (error out=w406:errorcluster, "Value"=w407:bool)  [unwired: 1 in, 1 out]
    n190 = case shown="True" w407 {
      tunnel: w406 -> [w410 w418]
      tunnel: [w411 w421] -> w404
      tunnel: w409 -> [_ w422]
      frame False {
        n191 = call "Stall Data Flow.vim"("value in"=w410, "milliseconds to wait"=u32 10) -> ("value out"=w411:errorcluster)  [unwired: 1 out]
      }
      frame True {
        w420 = 0 items=["standart", "extended"] ("type")
        w419 = u16 28 items=["1M"=20, "500K"=28, "250K"=284, "125K"=796, "100K"=17199, "50K"=18223, "20K"=21295, "10K"=26415, "5K"=32639] ("baud")
        n192 = call "PCAN_INIT.vi"("error in (no error)"=w418, "Msg Type"=w420, "BTR0BTR1"=w419) -> ("error out"=w417:errorcluster)  [unwired: 1 in, 7 out]
        n193 = for {
          N: 2 -> [_]
          tunnel: w422 -> [w430]
          shift-right: [w424] -> w415
          shift-left: w417 -> [w425]
          n194 = property on="Tx_DATA" class="Arr (strict)"() -> ("Value"=w427:u8[])  [unwired: 2 in, 2 out]
          n195 = property on="Tx_ID" class="DigNum (strict)"() -> ("Value"=w428:u32)  [unwired: 2 in, 2 out]
          n196 = Bundle By Name(cluster=w430, "ID"=w428, "aDATA"=w427, "LEN"=u8 8) -> (w429:T1)
          n197 = call "PCAN_WRITE.vi"("error in (no error)"=w425, "TPCANMsg"=w429) -> ("error out"=w424:errorcluster)  [unwired: 1 in, 8 out]
          n198 = Wait (ms)(milliseconds to wait=u32 100) -> ()  [unwired: 1 out]
        }
        n199 = call "Stall Data Flow.vim"("value in"=w415, "milliseconds to wait"=u32 100) -> ("value out"=w414:errorcluster)  [unwired: 1 out]
        n200 = while {
          shift-right: [w433] -> w421
          shift-left: w414 -> [w438]
          stop <- w431 stop-if-true
          n201 = call "PCAN_READ.vi"("error in (no error)"=w438) -> ("error out"=w437:errorcluster, "TPCANMsg"=w439:T1, "error"=w440:T4)  [unwired: 1 in, 7 out]
          n202 = case shown="0" w440 {
            selector: w440 -> [w449 _ _]
            tunnel: w439 -> [_ w459 _]
            tunnel: w437 -> [w450 w452 w460]
            tunnel: [w448 w451 w460] -> w435
            frame Default {
              n203 = call "PCAN_ERROR.vi"("error in (no error)"=w450, "Error Code"=w449) -> ("error out"=w448:errorcluster, "PCAN error"=w447:T5)  [unwired: 8 out]
              n204 = Wait (ms)(milliseconds to wait=u32 20) -> ()  [unwired: 1 out]
              n205 = call <vilib>:"Space Constant.vi"() -> ("String"=w441:string)
              n206 = Unbundle By Name(w447) -> ("Message"=w442:string)
              n207 = Get Date/Time String() -> (date string=w445:string, time string=w444:string)  [unwired: 3 out]
              n208 = Concatenate Strings(w445, w441, w444, w441, w442) -> (→"Last Error":string)
            }
            frame 0 {
              n209 = Unbundle By Name(w459) -> ("ID"=w458:u32, "aDATA"=w456:u8[])
              "CAN_ID" <- w458
              n210 = Equal?(x="Rx_ID", y=w458) -> (x = y?=w454:bool)
              n211 = Select(t=w456, s=w454, f=u8[] []) -> (s? t:f=w453:u8[])
              n212 = property on="Rx_DATA" class="Arr (strict)"(error in=w452, "Value"=w453) -> (error out=w451:errorcluster)  [unwired: 1 in, 1 out]
            }
            frame 32 {
              # "Wait if Buffer is empty"
              n213 = Wait (ms)(milliseconds to wait=u32 20) -> ()  [unwired: 1 out]
            }
          }
          n214 = call "Stall Data Flow.vim"("value in"=w435, "milliseconds to wait"=u32 10) -> ("value out"=w434:errorcluster)  [unwired: 1 out]
          n215 = property on="CAN_Tx" class="Bool (strict)"(error in=w434) -> (error out=w433:errorcluster, "Value"=w432:bool)  [unwired: 1 in, 1 out]
          n216 = Not(x=w432) -> (.not. x?=w431:bool)
        }
      }
    }
    n217 = property on="Stop" class="Bool (strict)"() -> ("Value"=w408:bool)  [unwired: 2 in, 2 out]
    n218 = call "PCAN_CLOSE.vi"("error in (no error)"=w404) -> ("error out"=w405:errorcluster)  [unwired: 10 out]
  }
  n219 = call <vilib>:"Simple Error Handler.vi"("error in (no error)"=w7) -> ("error out"=w6:errorcluster)  [unwired: 4 in, 4 out]
  n220 = Merge Errors(w6, w2) -> (w5:errorcluster)
  n221 = disable-structure shown="RUN_TIME_ENGINE==True" {
    disable-tunnel: w5 -> [_ _]
    frame condition #0 (active) {
    }
    frame condition #1 {
      # "Call Quit LabVIEW if running as a built application."
      n222 = Quit LabVIEW() -> ()  [unwired: 1 in]
    }
  }
